vi "Get Next Name from Attribute List.vi"(7 "element name (for errors)":string, 8 "error in":errorcluster, 9 "offset":i32, 11 "attribute list":string) -> (0 "error out":errorcluster, 1 "offset past name":i32, 2 "name":string)   [LabVIEW 2013]
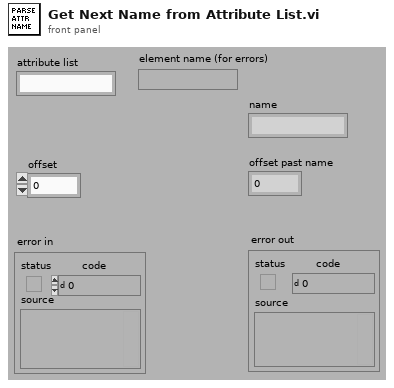
[diagram p1: front panel]
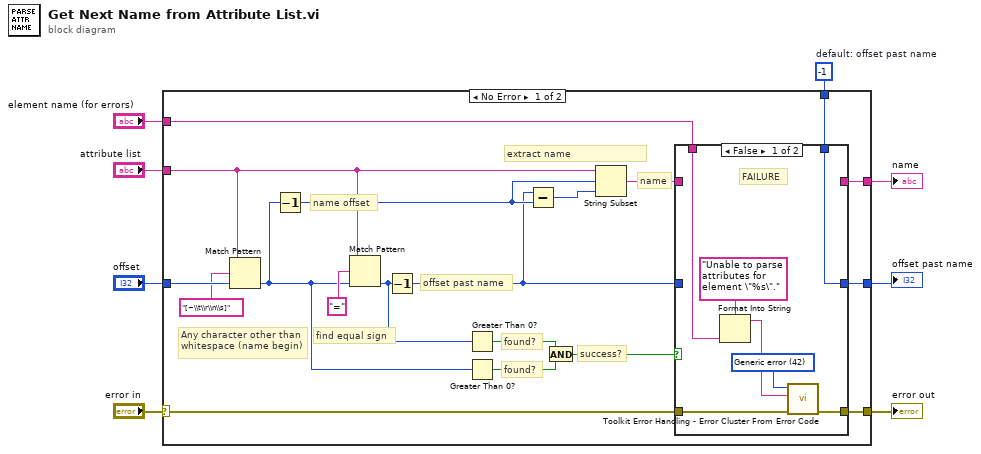
[diagram p0: block diagram]
diagram:
  w2 = -1  # default: offset past name
  n1 = case shown="No Error" "error in" {
    selector: "error in" -> [w12 w39]
    tunnel: [w14 w38] -> w8
    tunnel: "offset" -> [w25 _]
    tunnel: [w15 _] -> w6
    tunnel: "attribute list" -> [w22 _]
    tunnel: [w11 w39] -> w4
    tunnel: w2 -> [w10 w38]
    tunnel: "element name (for errors)" -> [w9 _]
    frame No Error {
      # "found?"
      # "found?"
      # "success?"
      # "extract name"
      # "name"
      # "offset past name"
      # "name offset"
      # "find equal sign"
      # "Any character other than whitespace (name begin)"
      n2 = Match Pattern(string=w22, regular expression="[~\\t\\r\\n\\s]", offset (0)=w25) -> (offset past match=w21:i32)  [unwired: 3 out]
      n3 = Decrement(x=w21) -> (x-1=w26:i32)
      n4 = Match Pattern(string=w22, regular expression="=", offset (0)=w21) -> (offset past match=w20:i32)  [unwired: 3 out]
      n5 = Decrement(x=w20) -> (x-1=w13:i32)
      n6 = Greater Than 0?(x=w20) -> (x > 0?=w19:bool)
      n7 = Greater Than 0?(x=w21) -> (x > 0?=w18:bool)
      n8 = Subtract(x=w13, y=w26) -> (x-y=w27:i32)
      n9 = And(x=w19, y=w18) -> (x .and. y?=w17:bool)
      n10 = String Subset(string=w22, offset (0)=w26, length (rest)=w27) -> (substring=w16:string)
      n11 = case shown="False" w17 {
        tunnel: [_ w37] -> w15
        tunnel: w16 -> [_ w37]
        tunnel: [w34 w36] -> w14
        tunnel: w13 -> [_ w36]
        tunnel: w12 -> [w33 w35]
        tunnel: [w32 w35] -> w11
        tunnel: w10 -> [w34 _]
        tunnel: w9 -> [w30 _]
        frame False {
          w31 = 42 items=["No error", "Argument error", "Memory is full", "Out of zone", "End of file", "File already open", "Generic file I/O error", "File not found", "File permission error", "Disk is full", "Duplicate path", "Too many files open", "System feature not enabled", "Resource file not found", "Cannot add resource", "Resource not found", "Image not found", "Image memory error", "Pen does not exist", "Config type invalid", "Config token not found", "Config parse error", "Config memory error", "Bad external code format", "Bad external code offset", "External code not present", "Null window", "Destroy window error", "Null menu", "Print aborted", "Bad print record", "Print driver error", "Windows error during printing", "Memory error during printing", "Print dialog error", "Generic print error", "Invalid device refnum", "Device not found", "Device parameter error", "Device unit error", "Cannot open device", "Device call aborted", "Generic error", "Cancelled by user", "Object ID too low", "Object ID too high", "Object not in heap", "Unknown heap", "Unknown object (invalid DefProc)", "Unknown object (DefProc not in table)", "Message out of range", "Invalid (null) method", "Unknown message", "Manager call not supported", "Bad address", "Network operation in progress", "Network operation timed out", "Connection is busy", "Network attribute not supported", "Network error", "Address in use", "System out of memory", "Connection aborted", "Connection refused", "Not connected", "Already connected", "Connection closed", "Initialization error (interapplication manager)", "Bad occurrence", "Wait on unbound occurrence handler", "Occurrence queue overflow", "Datalog type conflict", "Unused", "Unrecognized type (interapplication manager)", "Memory corrupt", "Failed to make temporary DLL", "Old CIN version", "Drag socket not found", "Failed to load drop-object", "Failed to register OLE object", "Failed to release OLE object", "Format specifier type mismatch", "Unknown format specifier", "Too few format specifiers", "Too many format specifiers", "Scan failed", "Newer CIN version", "Error converting to variant", "Runtime menu error", "Password tampered", "Variant attribute not found", "Incompatible variant data type", "Event data is not available", "Event Store is not present", "Occurrence is not found", "Event Queue is not created", "Event info is not available", "Refnum passed is NULL", "Error retrieving Class GUID", "Error retrieving CoClass GUID", "Error retrieving TypeLib GUID.", "Bad built application magic bytes.", "Specific driver is different from the specific driver associated with the Logical Name.", "There is no session opened to the class driver.", "Max Error", "MAX - Error with config objects", "MAX - Error loading configuration", "MAX - Group not supported"]
          # "FAILURE"
          n12 = Format Into String(format string="Unable to parse attributes for element \"%s\".", w30) -> (resulting string=w28:string)  [unwired: 2 in, 1 out]
          n13 = call "Toolkit Error Handling - Error Cluster From Error Code.vi"("error in"=w33, "error message (\"\")"=w28, "error code (0)"=w31) -> ("error out"=w32:errorcluster)  [unwired: 6 in]
        }
        frame True {
          # "SUCCESS"
        }
      }
    }
    frame Error {
    }
  }
  "offset past name" <- w8
  "name" <- w6
  "error out" <- w4
